vi "GeBitfieldList.vi"(0 "Data":T1) -> (14 "Array":string[](array[string]))   [LabVIEW 2017]
uses:
  Ctrl/Property.ctl
  Ctrl/PhysicalChannel.ctl
  Ctrl/Bitfield.ctl
  Ctrl/Register.ctl
  Ctrl/ScaleType.ctl
  Ctrl/Scale.ctl
  Ctrl/EnumValue.ctl
  Ctrl/Enum.ctl
  Ctrl/Caps.ctl
  Ctrl/Data.ctl
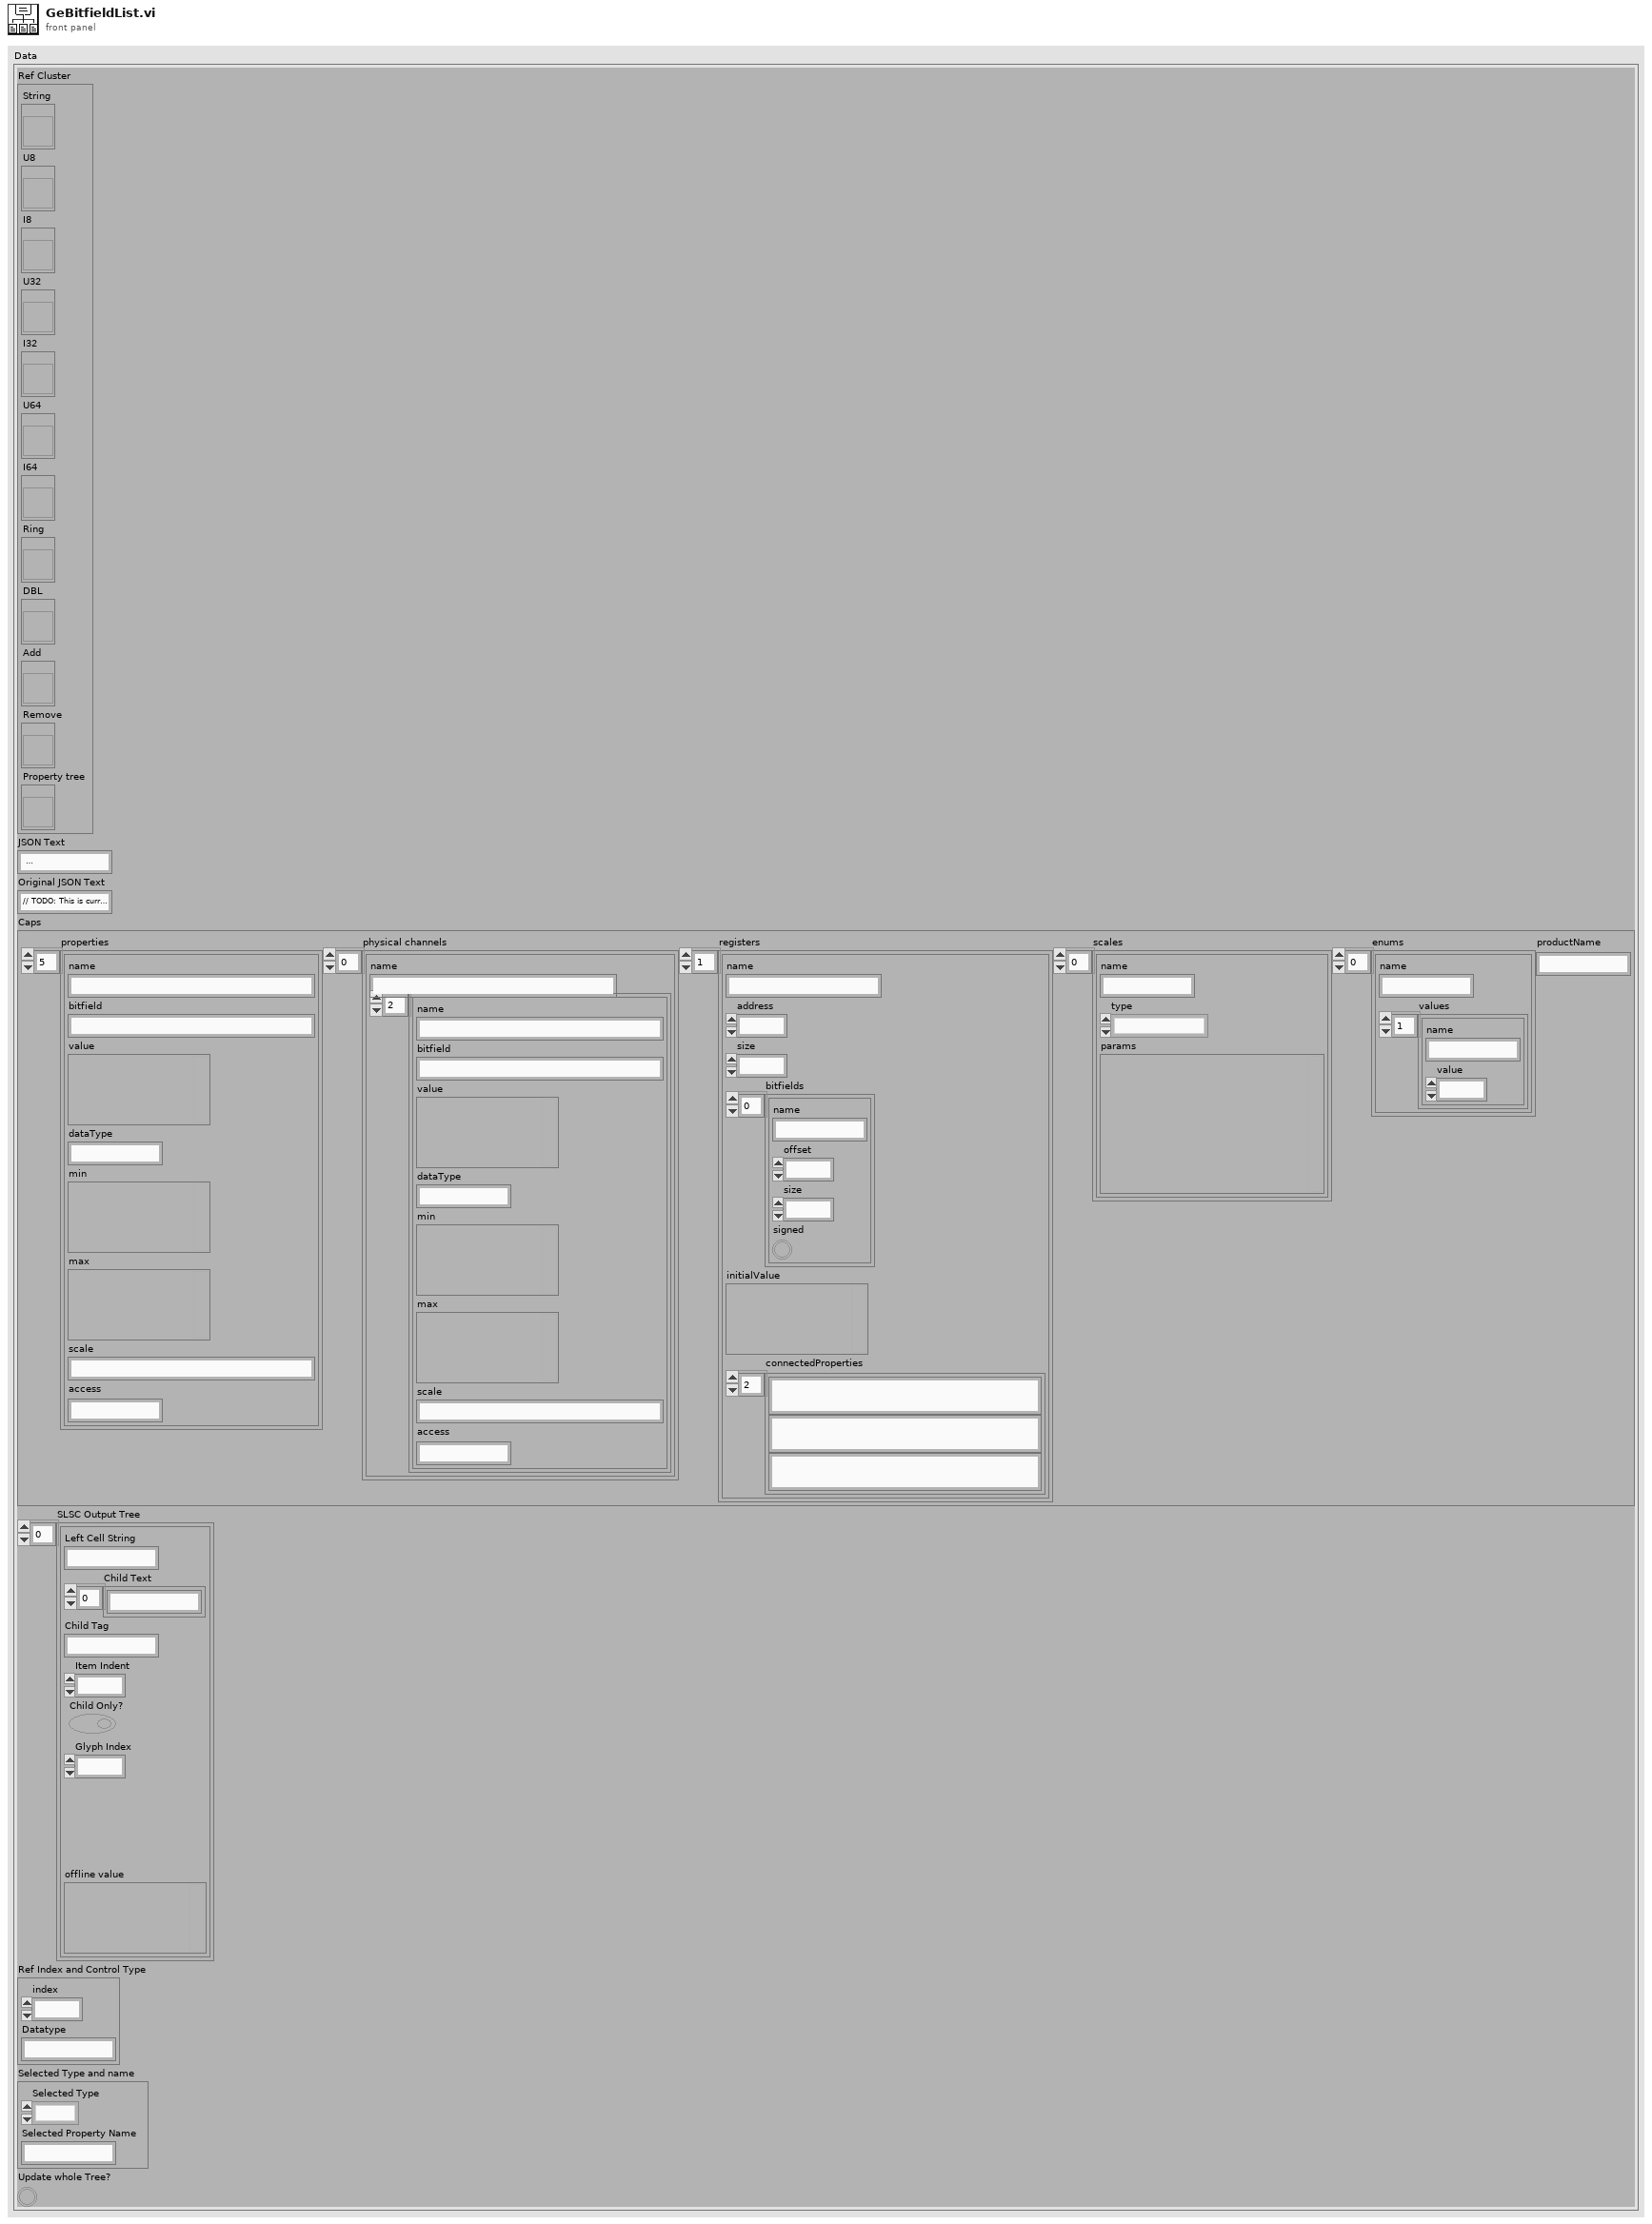
[diagram p1: front panel]
types:
  T1 = typedef "Data.ctl" = cluster{"Ref Cluster":cluster{"String":refnum<vi>, "U8":refnum<vi>, "I8":refnum<vi>, "U32":refnum<vi>, "I32":refnum<vi>, "U64":refnum<vi>, "I64":refnum<vi>, "Ring":refnum<vi>, "DBL":refnum<vi>, "Add":refnum<vi>, "Remove":refnum<vi>, "Property tree":refnum<vi>}, "JSON Text":string, "Original JSON Text":string, "Caps":T2, "SLSC Output Tree":cluster{"Left Cell String":string, "Child Text":string[], "Child Tag":string, "Item Indent":i32, "Child Only?":bool, "Glyph Index":i32, "offline value":variant}[], "Ref Index and Control Type":cluster{"index":i32, "Datatype":string}, "Selected Type and name":cluster{"Selected Type":enum16{"Property", "Physical Channel"}, "Selected Property Name":string}, "Update whole Tree?":bool}
  T2 = typedef "Caps.ctl" = cluster{"properties":T3[], "physical channels":T4[], "registers":T5[], "scales":T7[], "enums":T9[], "productName":string}
  T3 = typedef "Property.ctl" = cluster{"name":string, "bitfield":string, "value":variant, "dataType":string, "min":variant, "max":variant, "scale":string, "access":string}
  T4 = typedef "PhysicalChannel.ctl" = cluster{"name":string, "properties":T3[]}
  T5 = typedef "Register.ctl" = cluster{"name":string, "address":i32, "size":i32, "bitfields":T6[], "initialValue":variant, "connectedProperties":string[]}
  T6 = typedef "Bitfield.ctl" = cluster{"name":string, "offset":i32, "size":i32, "signed":bool}
  T7 = typedef "Scale.ctl" = cluster{"name":string, "type":T8, "params":variant}
  T8 = typedef "ScaleType.ctl" = enum16{"NoScale", "Table", "Polynomial", "Linear"}
  T9 = typedef "Enum.ctl" = cluster{"name":string, "values":T10[]}
  T10 = typedef "EnumValue.ctl" = cluster{"name":string, "value":i32}
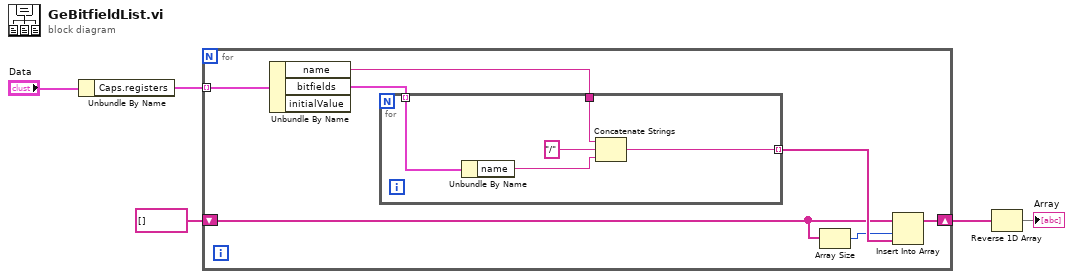
[diagram p0: block diagram]
diagram:
  n1 = Unbundle By Name("Data") -> ("Caps.registers"=w4:T5[])
  n2 = for {
    tunnel: w4 -> [w12] mode=indexing
    shift-right: [w9] -> w2
    shift-left: string[] [] -> [w7]
    n3 = Unbundle By Name(w12) -> ("name"=w10:string, "bitfields"=w11:T6[])  [unwired: 1 out]
    n4 = for {
      tunnel: w11 -> [w15] mode=indexing
      tunnel: w10 -> [w17]
      tunnel: [w13] -> w8 mode=indexing
      n5 = Unbundle By Name(w15) -> ("name"=w14:string)
      n6 = Concatenate Strings(w17, "/", w14) -> (w13:string)
    }
    n7 = Array Size(array=w7) -> (size(s)=w6:i32)
    n8 = Insert Into Array(array=w7, index=w6, new element=w8) -> (w9:string[])
  }
  n9 = Reverse 1D Array(array=w2) -> (reversed array=→"Array":string[])
